vi "Read RunningStats.vi"(8 "error in (no error)":errorcluster, 11 "HttpDownloadTask in":refnum<class "HttpDownloadTask.lvclass">) -> (0 "error out":errorcluster, 2 "RunningStats":T1, 3 "HttpDownloadTask out":refnum<class "HttpDownloadTask.lvclass">)   [LabVIEW 2018, in "HttpClient_NET.lvlib" / "HttpDownloadTask.lvclass"]
doc: "<b> </b> <b> </b>\nHttpClient_NET\nJustin Young - Viviota\nCopyright (c) 2021\nLicense: BSD"
uses:
  HttpDownloadTask.lvclass
  Types/DownloadStats_Cluster.ctl
  HttpDownloadTask.lvclass/HttpDownloadTask.ctl
  HttpClient_NET.lvlib
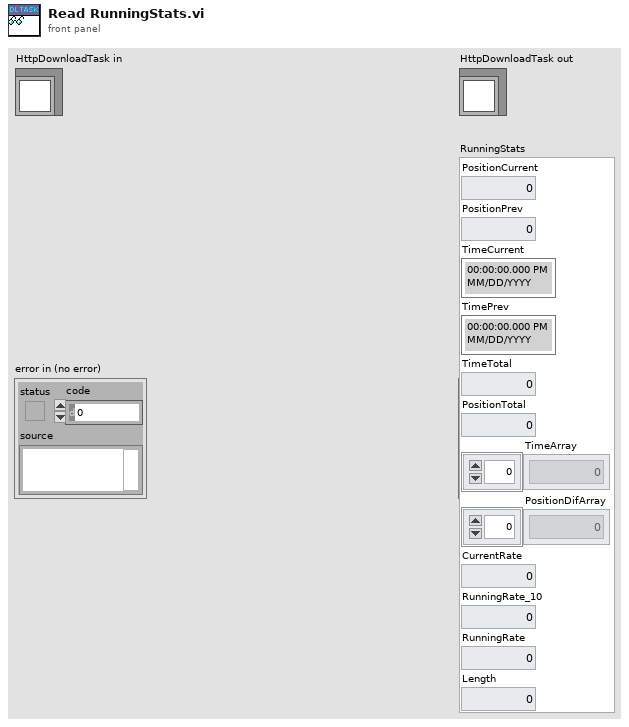
[diagram p1: front panel]
types:
  T1 = typedef "HttpClient_NET.lvlib/DownloadStats_Cluster.ctl" = cluster{"PositionCurrent":dbl, "PositionPrev":dbl, "TimeCurrent":timestamp, "TimePrev":timestamp, "TimeTotal":dbl, "PositionTotal":dbl, "TimeArray":dbl[], "PositionDifArray":dbl[], "CurrentRate":dbl, "RunningRate_10":dbl, "RunningRate":dbl, "Length":dbl}
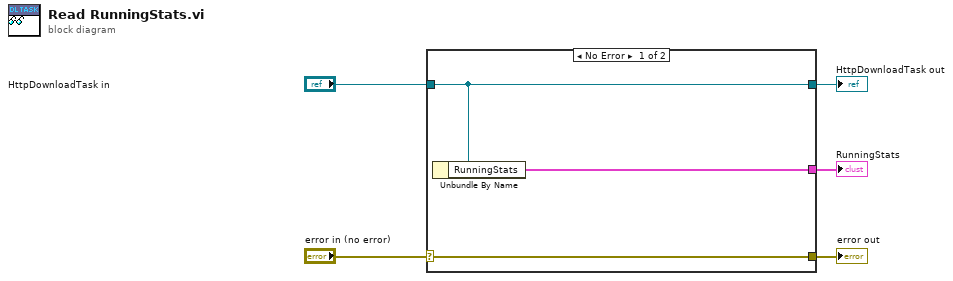
[diagram p0: block diagram]
diagram:
  n1 = case shown="No Error" "error in (no error)" {
    selector: "error in (no error)" -> [w8 w9]
    tunnel: [w8 w9] -> w4
    tunnel: [w7 w10] -> w2
    tunnel: "HttpDownloadTask in" -> [w7 w10]
    tunnel: [w6 _] -> w1
    frame No Error {
      n2 = Unbundle By Name(w7) -> ("RunningStats"=w6:T1)
    }
    frame Error {
    }
  }
  "error out" <- w4
  "HttpDownloadTask out" <- w2
  "RunningStats" <- w1
